vi "array vs var access speed.vi"() -> ()   [LabVIEW 2013]
panel:
  out "equal":bool
  out "RUN":dbl[](array[numeric])
  out "INIT":dbl[](array[numeric])
  in  "String length":i32=15
  in  "lookups":i32=10000
  in  "count":i32=150
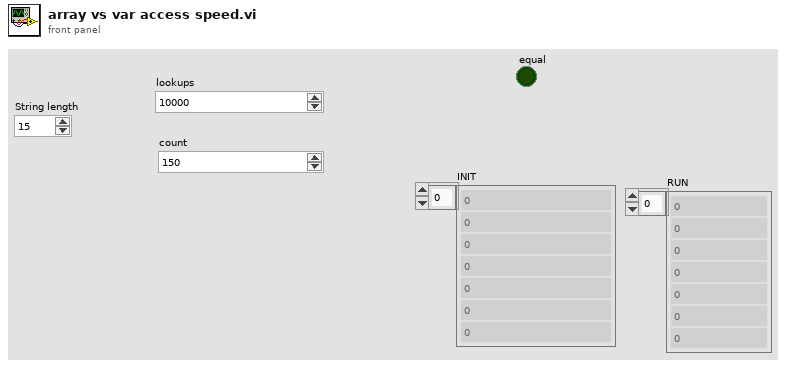
[diagram p1: front panel]
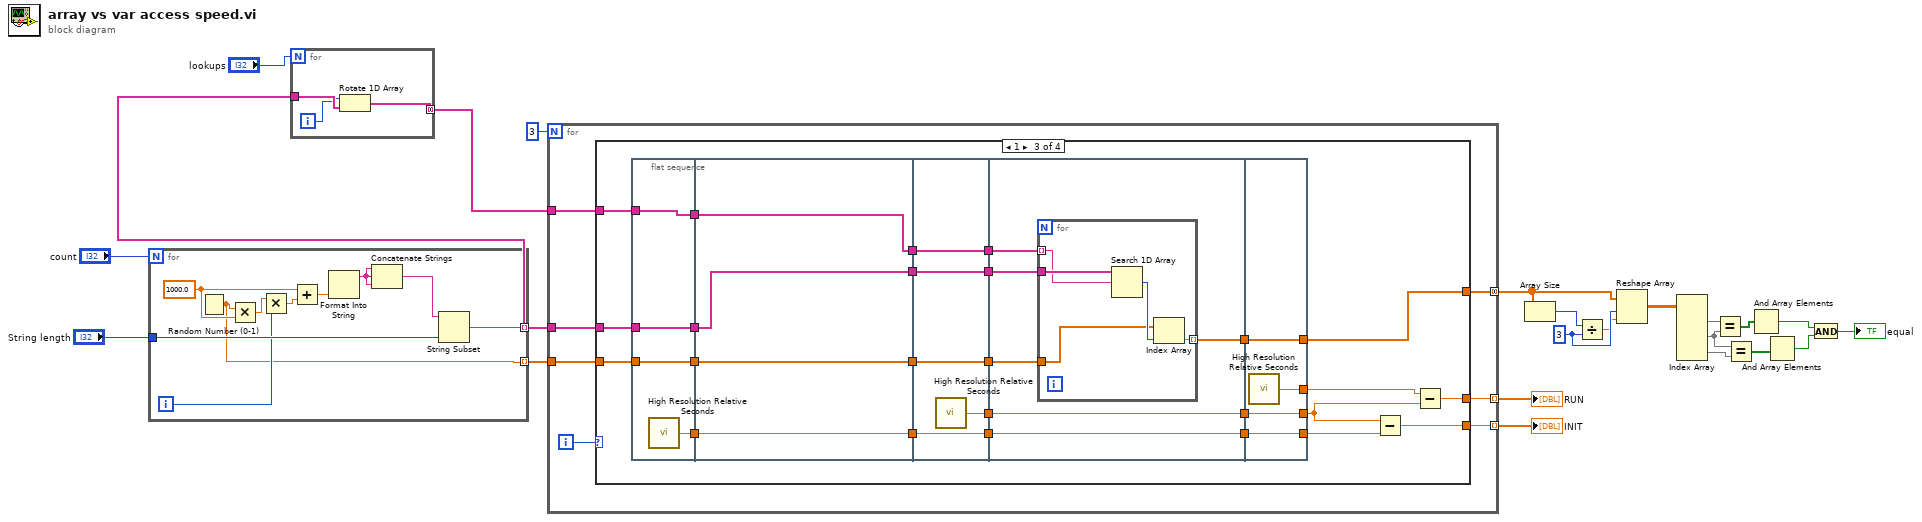
[diagram p0: block diagram]
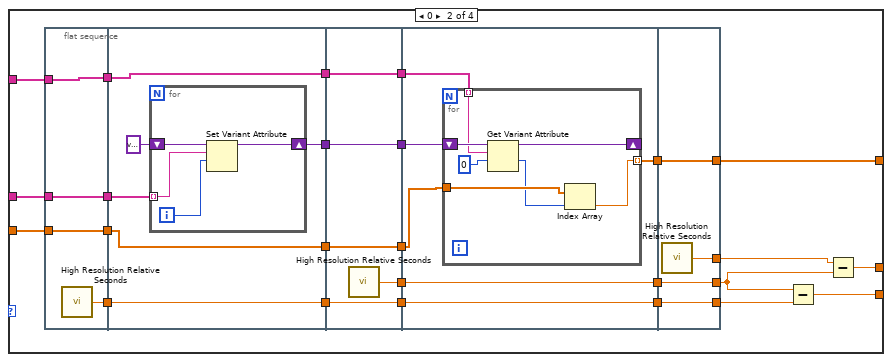
[diagram p3: hidden frame]
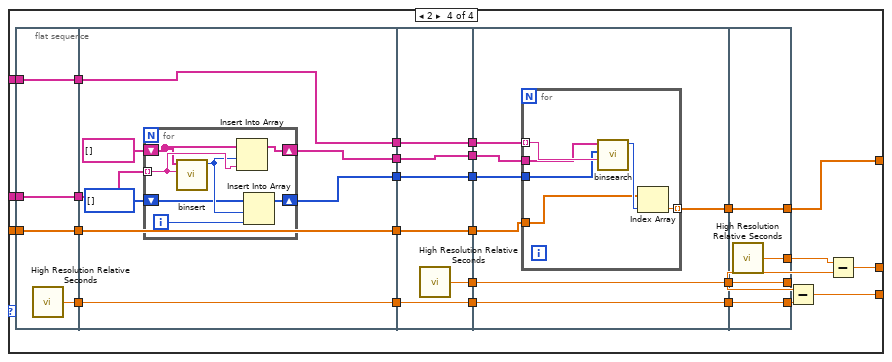
[diagram p4: hidden frame]
diagram:
  w11 = 3 ("y")
  n1 = for {
    N: "count" -> [_]
    tunnel: "String length" -> [w27]
    tunnel: [w23] -> w18 mode=indexing
    tunnel: [w25] -> w17 mode=indexing
    i -> [w24]
    w31 = 1000.0 ("y")
    n2 = Random Number (0-1)() -> (number: 0 to 1=w23:dbl)
    n3 = Multiply(x=w23, y=w31) -> (x*y=w32:dbl)
    n4 = Multiply(x=w32, y=w24) -> (x*y=w29:dbl)
    n5 = Add(x=w31, y=w29) -> (x+y=w30:dbl)
    n6 = Format Into String(w30) -> (resulting string=w28:string)  [unwired: 3 in, 1 out]
    n7 = Concatenate Strings(w28, w28, w28) -> (w26:string)
    n8 = String Subset(string=w26, length (rest)=w27) -> (substring=w25:string)  [unwired: 1 in]
  }
  n9 = for {
    N: "lookups" -> [_]
    tunnel: w17 -> [w35]
    tunnel: [w33] -> w16 mode=concatenating
    i -> [w34]
    n10 = Rotate 1D Array(1:w35, 2:w34) -> (0:w33:string[])
  }
  n11 = for {
    N: 3 -> [_]
    tunnel: [w41] -> w21 mode=indexing
    tunnel: [w40] -> w22 mode=indexing
    tunnel: w18 -> [w39]
    tunnel: w17 -> [w38]
    tunnel: [w37] -> w12 mode=concatenating
    tunnel: w16 -> [w36]
    i -> [w42]
    n12 = case shown="1" w42 {
      tunnel: [_ w58 w119 w174] -> w41
      tunnel: [_ w57 w118 w173] -> w40
      tunnel: w39 -> [_ w55 w116 w171]
      tunnel: w38 -> [_ w53 w114 w169]
      tunnel: [_ w48 w107 w166] -> w37
      tunnel: w36 -> [_ w45 w104 w161]
      frame Default {
      }
      frame 0 {
        n13 = flat-sequence {
          tunnel: [w71] -> w63
          tunnel: [w70] -> w56
          tunnel: w55 -> [w70]
          tunnel: [w69] -> w54
          tunnel: w53 -> [w69]
          tunnel: [w68] -> w46
          tunnel: w45 -> [w68]
          tunnel: [w77] -> w64
          tunnel: w63 -> [w77]
          tunnel: w56 -> [w72]
          tunnel: w54 -> [w75]
          tunnel: [w73] -> w51
          tunnel: [w74] -> w49
          tunnel: w46 -> [w73]
          tunnel: [w72] -> w43
          tunnel: [w86] -> w66
          tunnel: [w85] -> w65
          tunnel: w64 -> [w85]
          tunnel: [w84] -> w52
          tunnel: w51 -> [w84]
          tunnel: [w83] -> w50
          tunnel: w49 -> [w83]
          tunnel: [w82] -> w44
          tunnel: w43 -> [w82]
          tunnel: [w92] -> w67
          tunnel: w66 -> [w92]
          tunnel: w65 -> [w91]
          tunnel: [w91] -> w62
          tunnel: w52 -> [w90]
          tunnel: w50 -> [w89]
          tunnel: [w88] -> w47
          tunnel: w44 -> [w87]
          tunnel: [w103] -> w60
          tunnel: w67 -> [w102]
          tunnel: [w102] -> w59
          tunnel: [w101] -> w61
          tunnel: w62 -> [w101]
          tunnel: [w100] -> w48
          tunnel: w47 -> [w100]
          frame #0 {
            n14 = call <vilib>:"High Resolution Relative Seconds.vi"() -> ("relative seconds"=w71:dbl)
          }
          frame #1 {
            n15 = for {
              tunnel: w75 -> [w79] mode=indexing
              shift-right: [w81] -> w74
              shift-left: variant -> [w80]
              i -> [w78]
              n16 = Set Variant Attribute(Variant=w80, name=w79, value=w78) -> (Variant out=w81:variant)  [unwired: 1 in, 2 out]
            }
          }
          frame #2 {
            n17 = call <vilib>:"High Resolution Relative Seconds.vi"() -> ("relative seconds"=w86:dbl)
          }
          frame #3 {
            n18 = for {
              tunnel: w90 -> [w97] mode=indexing
              shift-right: [w98] -> _
              shift-left: w89 -> [w99]
              tunnel: [w94] -> w88 mode=indexing
              tunnel: w87 -> [w95]
              n19 = Get Variant Attribute(Variant=w99, name=w97, default value (empty Variant)=0) -> (duplicate Variant=w98:variant, value=w93:i32)  [unwired: 1 in, 2 out]
              n20 = Index Array(array=w95, index=w93) -> (element=w94:dbl)
            }
          }
          frame #4 {
            n21 = call <vilib>:"High Resolution Relative Seconds.vi"() -> ("relative seconds"=w103:dbl)
          }
        }
        n22 = Subtract(x=w59, y=w61) -> (x-y=w57:dbl)
        n23 = Subtract(x=w60, y=w59) -> (x-y=w58:dbl)
      }
      frame 1 {
        n24 = flat-sequence {
          tunnel: [w132] -> w124
          tunnel: [w131] -> w117
          tunnel: w116 -> [w131]
          tunnel: [w130] -> w115
          tunnel: w114 -> [w130]
          tunnel: [w129] -> w105
          tunnel: w104 -> [w129]
          tunnel: [w136] -> w125
          tunnel: w124 -> [w136]
          tunnel: w117 -> [w135]
          tunnel: w115 -> [w134]
          tunnel: [w133] -> w112
          tunnel: [w135] -> w110
          tunnel: [w134] -> w108
          tunnel: w105 -> [w133]
          tunnel: [w141] -> w127
          tunnel: [w140] -> w126
          tunnel: w125 -> [w140]
          tunnel: [w139] -> w113
          tunnel: w112 -> [w139]
          tunnel: [w138] -> w111
          tunnel: w110 -> [w138]
          tunnel: [w137] -> w109
          tunnel: w108 -> [w137]
          tunnel: [w147] -> w128
          tunnel: w127 -> [w147]
          tunnel: w126 -> [w146]
          tunnel: [w146] -> w123
          tunnel: w113 -> [w145]
          tunnel: w111 -> [w143]
          tunnel: w109 -> [w144]
          tunnel: [w142] -> w106
          tunnel: [w156] -> w121
          tunnel: w128 -> [w155]
          tunnel: [w155] -> w120
          tunnel: [w154] -> w122
          tunnel: w123 -> [w154]
          tunnel: [w153] -> w107
          tunnel: w106 -> [w153]
          frame #0 {
            n25 = call <vilib>:"High Resolution Relative Seconds.vi"() -> ("relative seconds"=w132:dbl)
          }
          frame #1 {
          }
          frame #2 {
            n26 = call <vilib>:"High Resolution Relative Seconds.vi"() -> ("relative seconds"=w141:dbl)
          }
          frame #3 {
            n27 = for {
              tunnel: w145 -> [w151] mode=indexing
              tunnel: w144 -> [w152]
              tunnel: [w149] -> w142 mode=indexing
              tunnel: w143 -> [w148]
              n28 = Search 1D Array(1D array=w152, element=w151) -> (index of element=w150:i32)  [unwired: 1 in]
              n29 = Index Array(array=w148, index=w150) -> (element=w149:dbl)
            }
          }
          frame #4 {
            n30 = call <vilib>:"High Resolution Relative Seconds.vi"() -> ("relative seconds"=w156:dbl)
          }
        }
        n31 = Subtract(x=w120, y=w122) -> (x-y=w118:dbl)
        n32 = Subtract(x=w121, y=w120) -> (x-y=w119:dbl)
      }
      frame 2 {
        n33 = flat-sequence {
          tunnel: [w187] -> w179
          tunnel: [w186] -> w172
          tunnel: w171 -> [w186]
          tunnel: [w185] -> w170
          tunnel: w169 -> [w185]
          tunnel: [w184] -> w162
          tunnel: w161 -> [w184]
          tunnel: [w195] -> w180
          tunnel: w179 -> [w195]
          tunnel: w172 -> [w194]
          tunnel: w170 -> [w192]
          tunnel: [w194] -> w167
          tunnel: [w193] -> w163
          tunnel: w162 -> [w193]
          tunnel: [w188] -> w159
          tunnel: [w190] -> w158
          tunnel: [w208] -> w182
          tunnel: [w207] -> w181
          tunnel: w180 -> [w207]
          tunnel: [w206] -> w168
          tunnel: w167 -> [w206]
          tunnel: [w205] -> w164
          tunnel: w163 -> [w205]
          tunnel: [w204] -> w160
          tunnel: w159 -> [w204]
          tunnel: w158 -> [w203]
          tunnel: [w203] -> w157
          tunnel: [w215] -> w183
          tunnel: w182 -> [w215]
          tunnel: w181 -> [w214]
          tunnel: [w214] -> w178
          tunnel: w168 -> [w211]
          tunnel: [w213] -> w165
          tunnel: w164 -> [w212]
          tunnel: w160 -> [w210]
          tunnel: w157 -> [w209]
          tunnel: [w225] -> w176
          tunnel: w183 -> [w224]
          tunnel: [w224] -> w175
          tunnel: [w223] -> w177
          tunnel: w178 -> [w223]
          tunnel: [w222] -> w166
          tunnel: w165 -> [w222]
          frame #0 {
            n34 = call <vilib>:"High Resolution Relative Seconds.vi"() -> ("relative seconds"=w187:dbl)
          }
          frame #1 {
            n35 = for {
              tunnel: w192 -> [w201] mode=indexing
              shift-right: [w202] -> w190
              shift-left: string[] [] -> [w200]
              shift-right: [w197] -> w188
              shift-left: i32[] [] -> [w196]
              i -> [w198]
              n36 = call "binsert.vi"("String"=w201, "strings"=w200) -> ("index"=w199:i32)  [unwired: 9 in]
              n37 = Insert Into Array(array=w200, index=w199, new element=w201) -> (w202:string[])
              n38 = Insert Into Array(array=w196, index=w199, new element=w198) -> (w197:i32[])
            }
          }
          frame #2 {
            n39 = call <vilib>:"High Resolution Relative Seconds.vi"() -> ("relative seconds"=w208:dbl)
          }
          frame #3 {
            n40 = for {
              tunnel: [w221] -> w213 mode=indexing
              tunnel: w212 -> [w220] mode=indexing
              tunnel: w211 -> [w218]
              tunnel: w210 -> [w217]
              tunnel: w209 -> [w216]
              n41 = call "binsearch.vi"("String"=w220, "indices"=w217, "strings"=w216) -> ("index"=w219:i32)  [unwired: 8 in]
              n42 = Index Array(array=w218, index=w219) -> (element=w221:dbl)
            }
          }
          frame #4 {
            n43 = call <vilib>:"High Resolution Relative Seconds.vi"() -> ("relative seconds"=w225:dbl)
          }
        }
        n44 = Subtract(x=w175, y=w177) -> (x-y=w173:dbl)
        n45 = Subtract(x=w176, y=w175) -> (x-y=w174:dbl)
      }
    }
  }
  "INIT" <- w22
  "RUN" <- w21
  n46 = Array Size(array=w12) -> (size(s)=w13:i32)
  n47 = Divide(x=w13, y=w11) -> (x/y=w10:dbl)
  n48 = Reshape Array(w12, w11, w10) -> (w9:dbl[][])
  n49 = Index Array(array=w9) -> (element #1=w8:dbl[], element #2=w7:dbl[], element #3=w6:dbl[])  [unwired: 6 in]
  n50 = Equal?(x=w8, y=w7) -> (x = y?=w4:bool[])
  n51 = Equal?(x=w7, y=w6) -> (x = y?=w5:bool[])
  n52 = And Array Elements(Boolean array=w4) -> (logical AND=w2:bool)
  n53 = And Array Elements(Boolean array=w5) -> (logical AND=w3:bool)
  n54 = And(x=w2, y=w3) -> (x .and. y?=→"equal":bool)
